vi "Timestamp_with_milliseconds_newFGGA.vi"(0 "Input Time":string="07:54:55.584 08/08/18") -> (4 "Output Time":string)   [LabVIEW 2014]
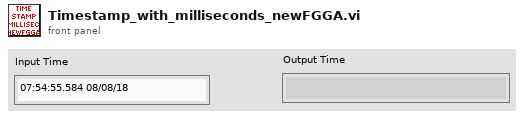
[diagram p1: front panel]
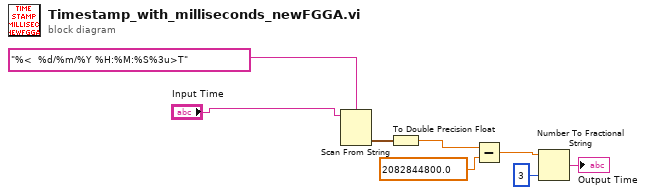
[diagram p0: block diagram]
diagram:
  n1 = Scan From String(format string="%<  %d/%m/%Y %H:%M:%S%3u>T", input string="Input Time") -> (output 1=w8:timestamp)  [unwired: 3 in, 3 out]
  n2 = To Double Precision Float(number=w8) -> (double precision float=w5:dbl)
  n3 = Subtract(x=w5, y=2082844800.0) -> (x-y=w4:dbl)
  n4 = Number To Fractional String(number=w4, precision (6)=i16 3) -> (F-format string=→"Output Time":string)  [unwired: 2 in]
